vi "DefaultFromINI.vi"(8 "error in (no error)":errorcluster, 11 "NHRDCModel":refnum<class "NHRDCPowerModel.lvclass">) -> (0 "error out":errorcluster, 3 "NHRDCModel":refnum<class "NHRDCPowerModel.lvclass">)   [LabVIEW 2018, in "AcPwrPlugins.lvlib" / "NHRDCPowerModel.lvclass"]
doc: "This VI loads the instruments' configuration previously stored on file."
uses:
  NHRDCPowerModel.lvclass
  F:/Program Files (x86)/National Instruments/LabVIEW 2018/user.lib/NIST/BaseClasses/BasePlugin_class/BasePlugin.lvclass
  F:/Projects/ICDAS/NistPluggableModules/AcPwr/AcPwrPlugins/AcPwrBaseClass/AcPwrBase.lvclass
  NHRDCPowerClass/TypeDefs/Device(s)Settings.ctl
  NHRDCPowerClass/TypeDefs/Modules.ctl
  NHRDCPowerClass/TypeDefs/Measurements.ctl
  <userlib>/NIST/BaseClasses/BasePlugin_class/BasePlugin.lvclass/BasePlugin.ctl
  <userlib>/NIST/BaseClasses/BasePlugin_class/Accessors/Read PluginIniFilePath.vi
  AcPwrBaseClass/AcPwrBase.lvclass
  <vilib>/Utility/config.llb/NI_LVConfig.lvlib
  NHRDCPowerClass/NHRDCPower.lvclass
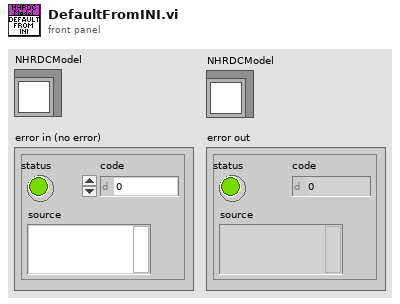
[diagram p1: front panel]
types:
  T1 = typedef "AcPwrPlugins.lvlib/NHRDCPower.lvclass/Measurements.ctl" = cluster{"Handle":string, "Name":string, "Enabled":bool, "Measurement Value":sgl, "Measurement Type":enum16{"Power", "Current", "Voltage"}}[]
  T2 = typedef "AcPwrPlugins.lvlib/NHRDCPower.lvclass/Device(s)Settings.ctl" = cluster{"MeasName":string, "Modules":T3}
  T3 = typedef "AcPwrPlugins.lvlib/NHRDCPower.lvclass/Modules.ctl" = cluster{"Handle":string, "Name":string, "id query (Yes)":bool, "reset device (Yes)":bool, "Connected":bool, "Initial Battery Detect Voltage (0)":dbl, "SafetySettings":cluster{"SetWatchDog?":bool, "Voltage (V)":dbl, "Current (A)":dbl, "Power (W)":dbl, "Voltage Delay (s)":dbl, "Current Delay (s)":dbl, "Power Delay (s)":dbl}, "Options String":string, "Aperture Time (s)":dbl, "operating state (Off)":i32, "OutputSettings":cluster{"Voltage (V)":dbl, "Current (A)":dbl, "Resistance (Ohms)":dbl, "Power (W)":dbl, "Enable Voltage":bool, "Enable Current":bool, "Enable Resistance":bool, "Enable Power":bool, "Macro After Step Delay  (s)":dbl, "Wait Value (V, A, W)":dbl, "Enable Wait":bool, "Wait on Value":i32}, "SlewRate":cluster{"Set Voltage Rate V/S":dbl, "Set Current Rate A/S":dbl, "Set Resistance Rate R/S":dbl, "Set Power Rate W/S":dbl}, "Macro":cluster{"Save Macro?":bool, "Load Macro From File?":bool, "Run Macro Continuously?":bool, "Use Macros?":bool, "Load Macro File Path":path, "Save Macro File Path":string}, "Regulation Gain (1=100%)":dbl, "UpdatingOntheFly":bool}[]
  T4 = typedef "NI_LVConfig.lvlib/Config Data RefNum.ctl" = refnum<k1>
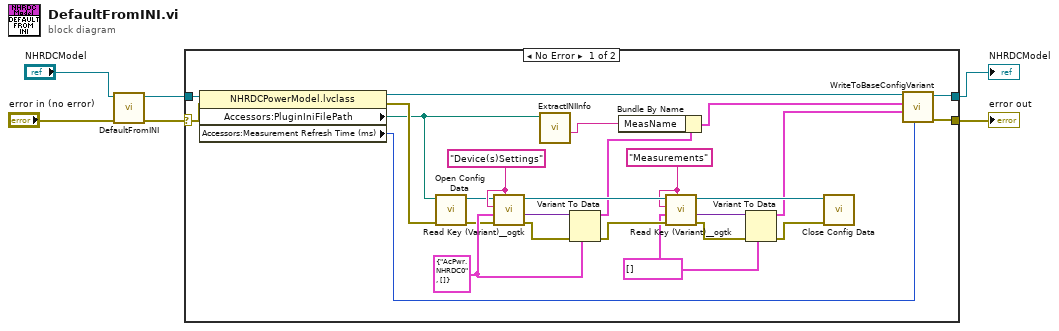
[diagram p0: block diagram]
diagram:
  n1 = call-parent "DefaultFromINI.vi"("error in (no error)"="error in (no error)", "AcPwrBase"="NHRDCModel") -> ("error out"=w4:errorcluster, "AcPwrBase"=w3:refnum<class "NHRDCPowerModel.lvclass">)  [unwired: 8 in]
  n2 = case shown="No Error" w4 {
    selector: w4 -> [w31 w33]
    tunnel: [w29 w34] -> w2
    tunnel: w3 -> [w32 w34]
    tunnel: [w30 w33] -> w1
    frame No Error {
      w17 = T1 [] ("Measurements")
      w18 = "Measurements" ("section")
      w25 = "Device(s)Settings" ("section")
      w26 = T2 {"MeasName"="AcPwr.NHRDC0", "Modules"=[]} ("NHRDC")
      n3 = property class="NHRDCPowerModel.lvclass"(reference=w32, error in=w31) -> (reference out=w27:refnum<class "NHRDCPowerModel.lvclass">, error out=w28:errorcluster, "Accessors:PluginIniFilePath"=w9:path, "Accessors:Measurement Refresh Time (ms)"=w11:u32)
      n4 = call <vilib>:"Open Config Data.vi"("error in (no error)"=w28, "configuration file path"=w9) -> ("error out"=w23:errorcluster, "refnum"=w24:T4)  [unwired: 7 in, 1 out]
      n5 = call <userlib>:"Read Key (Variant)__ogtk.vi"("section"=w25, "error in (no error)"=w23, "type"=w26, "key (optional)"=w25, "refnum"=w24) -> ("error out"=w22:errorcluster, "key-value"=w21:variant, "refnum out"=w19:T4)  [unwired: 3 in, 1 out]
      n6 = call "ExtractINIInfo.vi"("INI File Path"=w9) -> ("Plugin Name"=w8:string)  [unwired: 8 in, 2 out]
      n7 = Variant To Data(error in=w22, type=w26, Variant=w21) -> (data=w10:T2, error out=w20:errorcluster)
      n8 = Bundle By Name(cluster=w10, "MeasName"=w8) -> (w7:T2)
      n9 = call <userlib>:"Read Key (Variant)__ogtk.vi"("section"=w18, "error in (no error)"=w20, "type"=w17, "key (optional)"=w18, "refnum"=w19) -> ("error out"=w16:errorcluster, "key-value"=w15:variant, "refnum out"=w14:T4)  [unwired: 3 in, 1 out]
      n10 = Variant To Data(error in=w16, type=w17, Variant=w15) -> (data=w12:T1, error out=w13:errorcluster)
      n11 = call <vilib>:"Close Config Data.vi"("error in (no error)"=w13, "refnum"=w14) -> ()  [unwired: 8 in, 2 out]
      n12 = call-dynamic "WriteToBaseConfigVariant.vi"("Measurement Refresh Time (ms)"=w11, "Meas"=w12, "Config"=w7, "NHRDCModel in"=w27) -> ("error out"=w30:errorcluster, "NHRDCModel out"=w29:refnum<class "NHRDCPowerModel.lvclass">)  [unwired: 6 in]
    }
    frame Error {
    }
  }
  "error out" <- w1
  "NHRDCModel" <- w2
